vi "Arret Urgence.vi"() -> (0 "error out":errorcluster)   [LabVIEW 2013]
panel:
  in  "error in (no error)":errorcluster
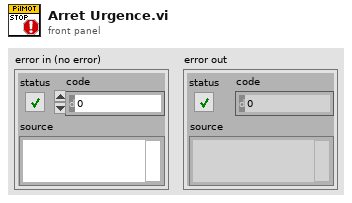
[diagram p1: front panel]
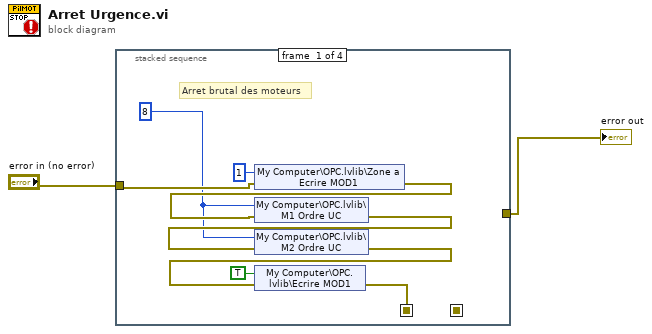
[diagram p0: block diagram]
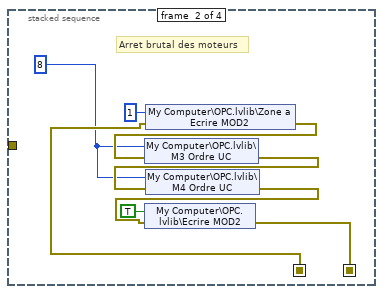
[diagram p2: hidden frame]
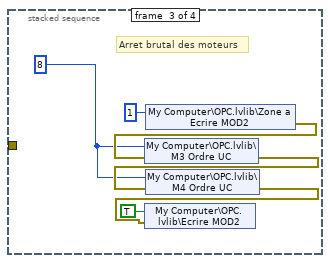
[diagram p3: hidden frame]
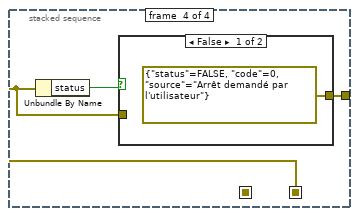
[diagram p4: hidden frame]
diagram:
  n1 = stacked-sequence {
    seq-local: [_ w18 _ _] -> [_ _ _ w25]
    seq-local: [w5 _ _ _] -> [_ w17 _ _]
    tunnel: "error in (no error)" -> [w9 _ _ _]
    tunnel: [_ _ _ w26] -> w1
    frame #0 {
      w4 = u16 8 ("Axe1_OrdreUC")
      # "Arret brutal des moteurs"
      n2 = shared-variable "My Computer\\OPC.lvlib\\Zone a Ecrire MOD1"(u16 1 ("Zone à Ecrire Module 1"), error in=w9) -> (error out=w8:errorcluster)
      n3 = shared-variable "My Computer\\OPC.lvlib\\M1 Ordre UC"(w4, error in=w8) -> (error out=w7:errorcluster)
      n4 = shared-variable "My Computer\\OPC.lvlib\\M2 Ordre UC"(w4, error in=w7) -> (error out=w6:errorcluster)
      n5 = shared-variable "My Computer\\OPC.lvlib\\Ecrire MOD1"(TRUE ("Ecrire Module 1"), error in=w6) -> (error out=w5:errorcluster)
    }
    frame #1 {
      w12 = u16 8 ("Axe3_OrdreUC")
      # "Arret brutal des moteurs"
      n6 = shared-variable "My Computer\\OPC.lvlib\\Zone a Ecrire MOD2"(u16 1 ("Zone à Ecrire Module2"), error in=w17) -> (error out=w15:errorcluster)
      n7 = shared-variable "My Computer\\OPC.lvlib\\M3 Ordre UC"(w12, error in=w15) -> (error out=w14:errorcluster)
      n8 = shared-variable "My Computer\\OPC.lvlib\\M4 Ordre UC"(w12, error in=w14) -> (error out=w13:errorcluster)
      n9 = shared-variable "My Computer\\OPC.lvlib\\Ecrire MOD2"(TRUE ("Ecrire Module2"), error in=w13) -> (error out=w18:errorcluster)
    }
    frame #2 {
      w20 = u16 8 ("Axe3_OrdreUC")
      # "Arret brutal des moteurs"
      n10 = shared-variable "My Computer\\OPC.lvlib\\Zone a Ecrire MOD2"(u16 1 ("Zone à Ecrire Module2")) -> (error out=w23:errorcluster)  [unwired: 1 in]
      n11 = shared-variable "My Computer\\OPC.lvlib\\M3 Ordre UC"(w20, error in=w23) -> (error out=w22:errorcluster)
      n12 = shared-variable "My Computer\\OPC.lvlib\\M4 Ordre UC"(w20, error in=w22) -> (error out=w21:errorcluster)
      n13 = shared-variable "My Computer\\OPC.lvlib\\Ecrire MOD2"(TRUE ("Ecrire Module2"), error in=w21) -> ()  [unwired: 1 out]
    }
    frame #3 {
      n14 = Unbundle By Name(w25) -> ("status"=w27:bool)
      n15 = case shown="False" w27 {
        tunnel: [errorcluster {"status"=FALSE, "code"=0, "source"="Arrêt demandé par l'utilisateur"} ("error out") w29] -> w26
        tunnel: w25 -> [_ w29]
        frame False {
        }
        frame True {
        }
      }
    }
  }
  "error out" <- w1
